vi "Encoder Test.vi"() -> ()   [LabVIEW 2016]
panel:
  out "Right Value":i32
  out "Left  Value":i32
  in  "stop":bool
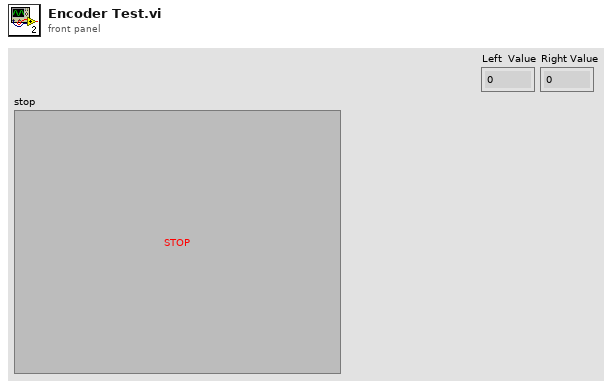
[diagram p1: front panel]
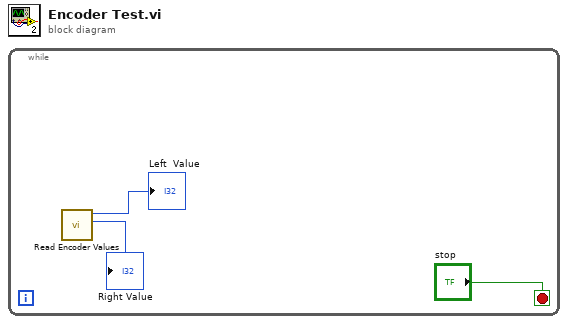
[diagram p0: block diagram]
diagram:
  n1 = while {
    stop <- "stop" stop-if-true
    n2 = call "Read Encoder Values.vi"() -> ("Right Value"=→"Right Value":i32, "Left  Value"=→"Left  Value":i32)  [unwired: 10 in]
  }
